vi "ADC Data capture and Process Original - Copy.vi"(0 "ADC Output Read Method":T2(ring)=enum."Read .dat file", 1 "Select the Tab to project":T1(ring)=enum."ADC Sine", 2 "ADC Input":enum16{"Sine Wave", "Ramp / Triangle"}(ring), 3 "No.of samples(SNR)":i32=4096, 4 "Resolution":i32=12, 5 "active edge":i32(ring)=10280, 6 "Inputs for Dyanmic para":T9={"Fundamental Frequency"=100000.0, "Sampling Frequncy"=3999610.0, "No of Harmonics"=9, "Window"=enum."7 Term B-Harris", "Blackman (fundamental power) bins)"=1.0}, 7 "Samples per Channel":i32=4096 caption="No.of Samples(capture)", 8 "Oversampling":bool, 9 "Oversampling ratio":i32, 10 "Drop LSB":bool, 11 "Save data":T15, 12 "Waveform":i64[](array[numeric]), 13 "Path to Read":path=path "C/Users/a0230227/Desktop/save.dat", 14 "Start & Stop Bit":cluster{"Start":i32, "Stop":i32}={"Start"=40, "Stop"=4055}, 15 "length":i32=4096, 17 "Set_Freq":dbl=100017.0, 24 "path to save":T14={"Path to Save plot"=path "D/Tenor_176P/DYN_PAR_C004/DAT/D001_TEMPP30C_VDD1.2_VDDA3.3_16B_SE_ADCA__vicA_aggX_PLT_CAP_200821_1740_33.jpg", "Path to Raw Data plot"=path "D/Tenor_176P/DYN_PAR_C004/DAT/D001_TEMPP30C_VDD1.2_VDDA3.3_16B_SE_ADCA__vicA_aggX_RAW_DAT_200821_1740_33.csv"}) -> (18 "Min Max":T4, 19 "detected Throughput":dbl, 20 "output cluster":T7, 21 "Dynamic Parameters":T8, 22 "max code":ext, 23 "min code":ext, 25 "Valid Capture":bool)   [LabVIEW 2019] (continued)
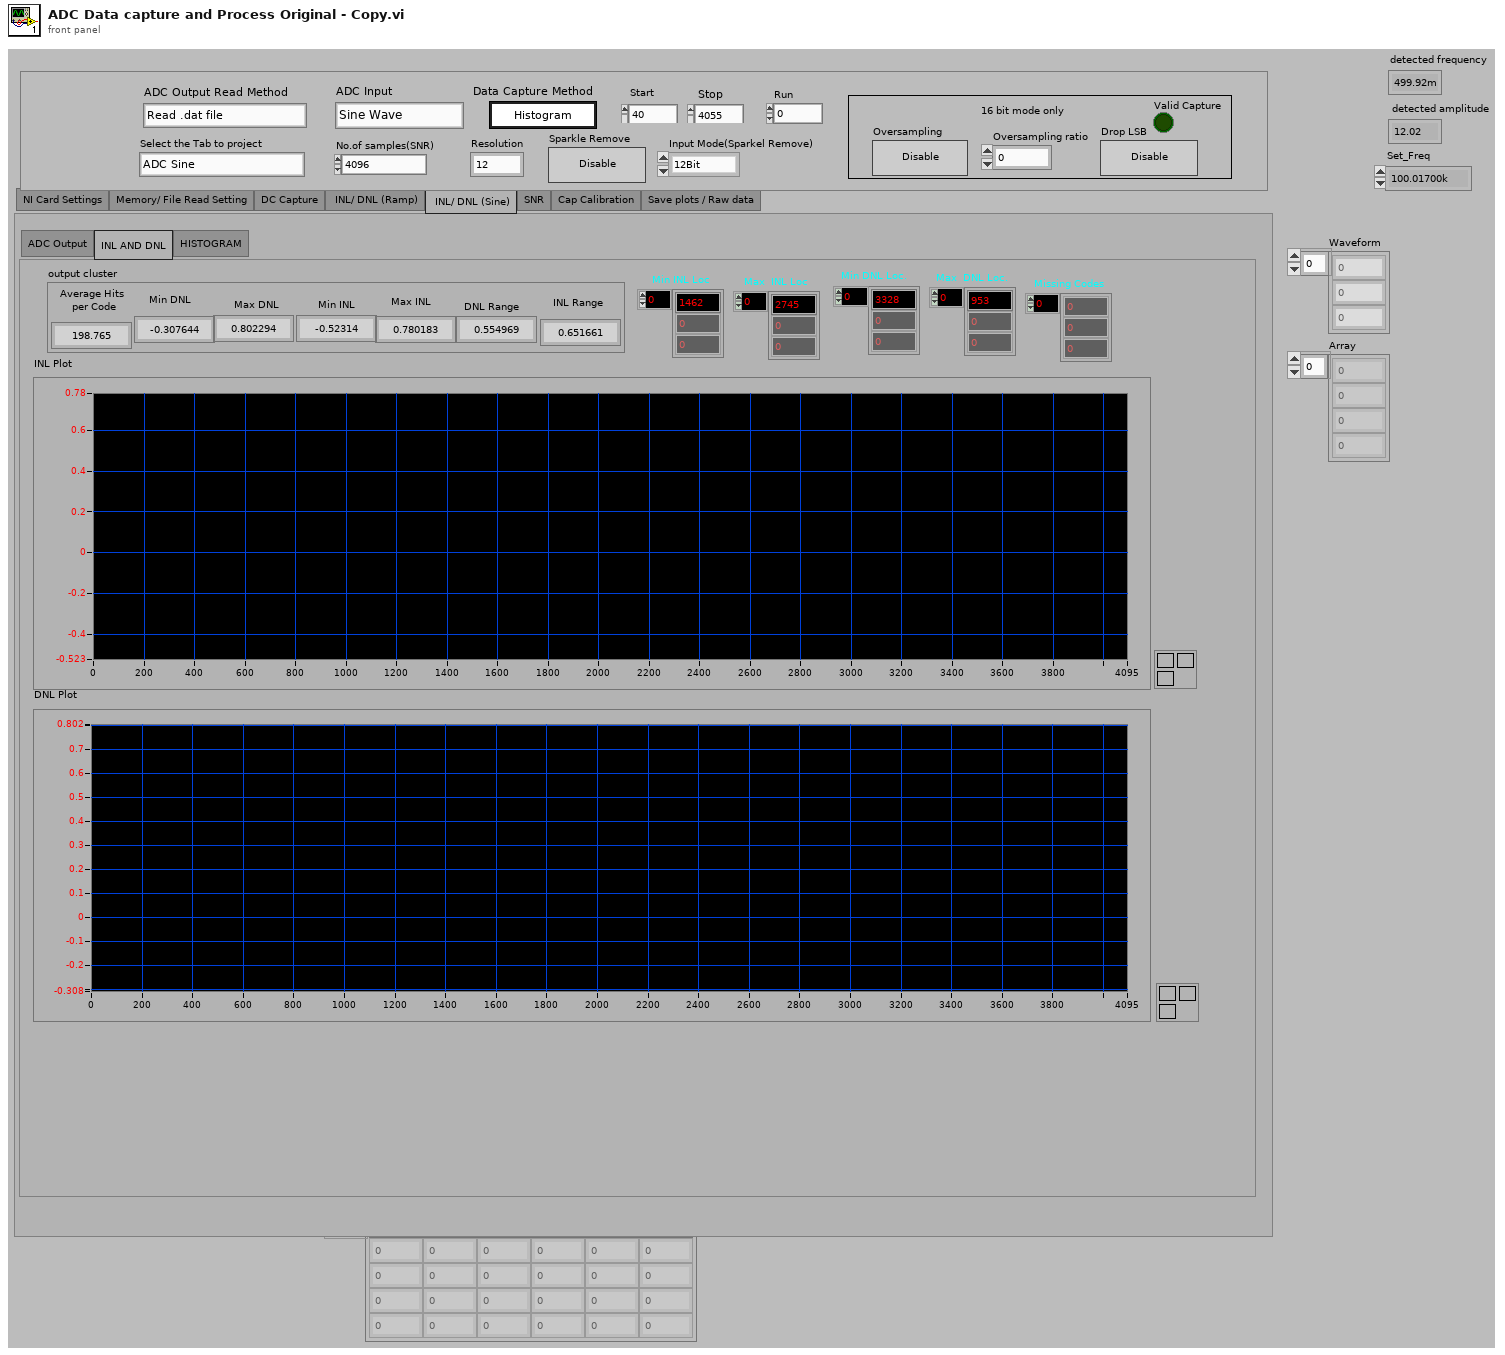
[diagram p1: front panel]
types:
  T1 = enum32{"NI Card Settings", "Memory Read Setting", "DC Capture", "ADC Ramp", "ADC Sine", "SNR", "Cap Calibration"}
  T2 = enum32{"Read from Memory", "Read .dat file", "NI Card Capture", "None"}
  T3 = enum32{"NI Card Settings", "Memory/ File Read Setting", "DC Capture", " INL/ DNL (Ramp)", " INL/ DNL (Sine)", "SNR", "Cap Calibration", "Save plots / Raw data"}
  T4 = cluster{"Min":dbl, "Max":dbl, "delta":dbl, "Average Code":dbl, "Standard Deviation":dbl}
  T5 = cluster{"Min INL":dbl, "Max INL":dbl, "Min DNL":dbl, "Max DNL":dbl, "INL Range":dbl, "DNL Range":dbl, "Avg Hits/Code":dbl}
  T6 = enum32{"ADC Output", "TRIMMED DATA", "INL AND DNL", "HISTOGRAM"}
  T7 = cluster{"Average Hits \nper Code ":dbl, "Min DNL":dbl, "Min INL":dbl, "Max INL":dbl, "Max DNL":dbl, "DNL Range":dbl, "INL Range":dbl}
  T8 = cluster{"SNR":dbl, "SNRD":dbl, "THD":dbl, "ENOB (SNRD)":dbl, "SFDR":dbl, "ENOB (SNR)":dbl, "Noise Power":dbl, "Signal power":dbl}
  T9 = cluster{"Fundamental Frequency":dbl, "Sampling Frequncy":dbl, "No of Harmonics":u8, "Window":enum16{"None ", "Hanning", "Hamming", "Blackman-Harris", "Exact Blackman", "Blackman", "Flat Top", "4 Term B-Harris ", "7 Term B-Harris"}, "Blackman (fundamental power) bins)":dbl}
  T10 = enum32{"ADC Output", "FFT Magnitude plot", " FFT plot"}
  T11 = cluster{"Ideal Power Bin":dbl, "Actual Power Bin":dbl, "Signal Strength (dB)":dbl}
  T12 = cluster{"ADC Reference(V)":dbl, "Bin Width":dbl, "PSRR/ CMRR  ":bool}
  T13 = cluster{"Fundamental Frequnecy (Calculated)":dbl, "Harmonic Frequencies":dbl[], "Harmonic Amplitudes":dbl[]}
  T14 = cluster{"Path to Save plot":path, "Path to Raw Data plot":path}
  T15 = cluster{"Save INL/DNL Plot(Ramp)":bool, "Save SNR Plot":bool, "Save INL/DNL Plot(Sine)":bool, "Save INL/DNL Raw Data(Ramp)":bool, "Save SNR Raw Data":bool, "Save INL/DNL Raw Data(Sine)":bool, "Save DC Raw data":bool, "Save  Raw Data(Sine)":bool}
  T16 = enum16{"Initialize", "Read output", "Post process", "Cap Calib", "Save data", "Exit"}
  T17 = cluster{"Average Hits \nper Code ":dbl, "Min\nDNL":dbl, dbl, dbl, "Max\nDNL":dbl, dbl, dbl}
  T18 = enum16{"None ", "Hanning", "Hamming", "Blackman-Harris", "Exact Blackman", "Blackman", "Flat Top", "4 Term B-Harris ", "7 Term B-Harris"}
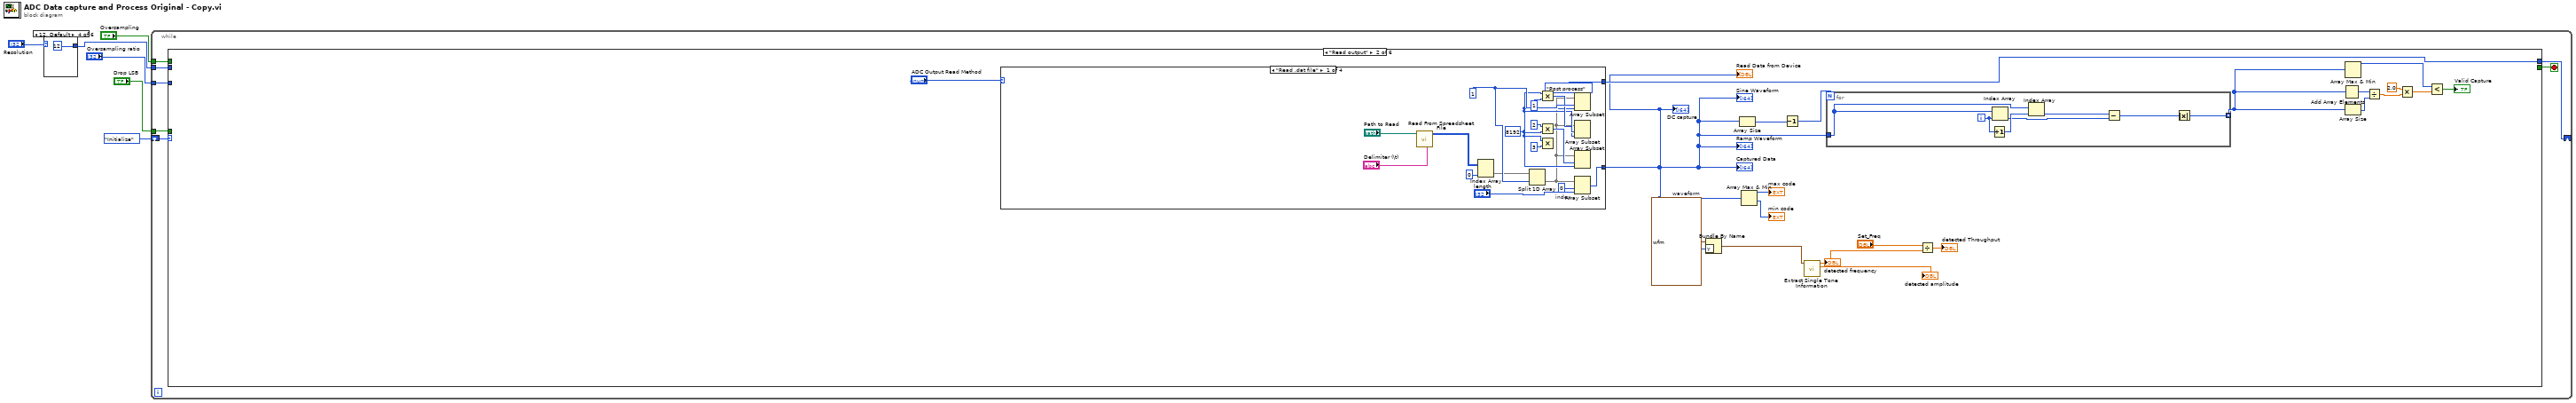
[diagram p0: block diagram]
diagram:
  n1 = case shown="12, Default" "Resolution" {
    tunnel: [18 16 14 12 10 8] -> w5
    frame 18 {
    }
    frame 16 {
    }
    frame 14 {
    }
    frame 12, Default {
    }
    frame 10 {
    }
    frame 8 {
    }
  }
  n2 = while {
    shift-right: [w18] -> _
    shift-left: T16."Initialize" -> [w19]
    tunnel: w5 -> [w16]
    tunnel: "Oversampling" -> [w15]
    tunnel: "Drop LSB" -> [w14]
    tunnel: "Oversampling ratio" -> [w13]
    stop <- w17 stop-if-true
    n3 = case shown="\"Read output\"" w19 {
      tunnel: [T16."Read output" w42 w125 T16."Save data" T16."Exit" _] -> w18
      tunnel: [_ _ _ _ _ TRUE] -> w17
      tunnel: w16 -> [_ _ w132 _ _ _]
      tunnel: w15 -> [_ _ w122 _ _ _]
      tunnel: w14 -> [_ _ w124 _ _ _]
      tunnel: w13 -> [_ _ w123 _ _ _]
      frame "Initialize", Default {
        n4 = local read "No.of samples(SNR)"() -> (w20:i32)
        n5 = local write "Samples per Channel"(w20) -> ()
      }
      frame "Read output" {
        w27 = waveform(i64) {"t0"=timestamp(0 s since 1904-01-01), "dt"=1.0, "Y"=[]}  # waveform
        n6 = case shown="\"Read .dat file\"" "ADC Output Read Method" {
          tunnel: [w52 _ w71 "Waveform"] -> w28
          tunnel: [T16."Post process" _ T16."Post process" T16."Post process"] -> w42
          frame "Read .dat file" {
            w51 = 0  # index
            w57 = 8192 ("index")
            w62 = 1 ("index")
            n7 = call-poly <vilib>:"Read From Spreadsheet File.vi"("delimiter (\\t)"="Delimiter (\\t)", "file path (dialog if empty)"="Path to Read") -> ("all rows"=w64:i64[][])  [unwired: 5 in, 4 out]
            n8 = Index Array(array=w64, index (col)=0 ("disabled index (col)")) -> (element=w55:i64[])  [unwired: 1 in]
            n9 = Split 1D Array(array=w55, index=w62) -> (second subarray=w53:i64[])  [unwired: 1 out]
            n10 = Multiply(x=w57, y=1) -> (x*y=w60:i32)
            n11 = Multiply(x=2 ("y"), y=w57) -> (x*y=w58:i32)
            n12 = Multiply(x=w57, y=3) -> ()  [unwired: 1 out]
            n13 = Array Subset(array=w53, index=w62, length=w57) -> ()  [unwired: 1 out]
            n14 = Array Subset(array=w53, index=w60, length=w57) -> ()  [unwired: 1 out]
            n15 = Array Subset(array=w53, index=w58, length=w57) -> ()  [unwired: 1 out]
            n16 = Array Subset(array=w53, index=w51, length="length") -> (w52:i64[])
          }
          frame "None" {
          }
          frame "NI Card Capture", Default {
            n17 = case shown="\"Sine Wave\", Default" "ADC Input" {
              tunnel: "Port" -> [w88 w108]
              tunnel: "Source" -> [w87 w107]
              tunnel: "Rate" -> [w86 w106]
              tunnel: "Timeout" -> [w85 w105]
              tunnel: [_ w103] -> w70
              tunnel: [w81 w104] -> w71
              tunnel: "No.of samples(SNR)" -> [w84 w102]
              tunnel: "Samples per Channel" -> [w82 w101]
              tunnel: "Sparkle Remove" -> [w80 _]
              tunnel: "active edge" -> [w79 w99]
              frame "Sine Wave", Default {
                n18 = disable-structure shown="Disabled" {
                  disable-tunnel: w88 -> [w98 _]
                  disable-tunnel: w87 -> [w97 _]
                  disable-tunnel: w86 -> [w96 _]
                  disable-tunnel: w85 -> [w95 _]
                  disable-tunnel: w84 -> [w94 _]
                  disable-tunnel: FALSE ("Histogram Capture Method SNR") -> [w93 _]
                  disable-tunnel: w82 -> [w92 _]
                  disable-tunnel: [w91 _] -> w81
                  disable-tunnel: w80 -> [w90 _]
                  disable-tunnel: w79 -> [w89 _]
                  frame Disabled {
                    n19 = call "DATA_CAPTURE_SNR.vi"("Port"=w98, "Source"=w97, "No. of samples to process"=w94, "Samples per Channel"=w92, "Rate"=w96, "active edge"=w89, "timeout"=w95, "Histogram Capture Method SNR"=w90, "NI card Cont/Single Capture"=w93) -> ("Waveform"=w91:u32[])  [unwired: 5 in, 5 out]
                  }
                  frame Enabled {
                  }
                }
              }
              frame "Ramp / Triangle" {
                n20 = disable-structure shown="Disabled" {
                  disable-tunnel: w108 -> [w119 _]
                  disable-tunnel: w107 -> [w118 _]
                  disable-tunnel: w106 -> [w117 _]
                  disable-tunnel: w105 -> [w116 _]
                  disable-tunnel: [w115 _] -> w104
                  disable-tunnel: [w114 _] -> w103
                  disable-tunnel: w102 -> [w113 _]
                  disable-tunnel: w101 -> [w111 _]
                  disable-tunnel: FALSE ("Histogram Capture Method SNR") -> [w110 _]
                  disable-tunnel: w99 -> [w109 _]
                  frame Disabled {
                    n21 = call "DATA_CAPTURE_SNR.vi"("Port"=w119, "Source"=w118, "No. of samples to process"=w113, "Samples per Channel"=w111, "Rate"=w117, "active edge"=w109, "timeout"=w116, "Histogram Capture Method SNR"=w110, "NI card Cont/Single Capture"=FALSE ("Histogram Capture Method SNR")) -> ("Waveform"=w115:u32[], "Trimmed Wave"=w114:u32[])  [unwired: 5 in, 4 out]
                  }
                  frame Enabled {
                  }
                }
              }
            }
            "Trimmed Wave" <- w70
          }
          frame "Read from Memory" {
          }
        }
        "Ramp Waveform" <- w28
        "Sine Waveform" <- w28
        "Read Data from Device" <- w28
        "Captured Data" <- w28
        "DC capture" <- w28
        n22 = Bundle By Name(cluster=w27, "Y"=w28) -> (w26:waveform(i64))
        n23 = Array Size(array=w28) -> (size(s)=w38:i32)
        n24 = Array Max & Min(array=w28) -> (max value=→"max code":i64, min value=→"min code":i64)  [unwired: 2 out]
        n25 = Decrement(x=w38) -> (x-1=w37:i32)
        n26 = call-poly <vilib>:"Extract Single Tone Information.vi"("time signal in"=w26) -> ("detected amplitude"=→"detected amplitude":dbl, "detected frequency"=w23:dbl)  [unwired: 5 in, 4 out]
        "detected frequency" <- w23
        n27 = for {
          N: w37 -> [_]
          tunnel: w28 -> [w49]
          tunnel: [w43] -> w35 mode=indexing
          i -> [w47]
          n28 = Increment(x=w47) -> (x+1=w48:i32)
          n29 = Index Array(array=w49, index=w47) -> (element=w45:i64)
          n30 = Index Array(array=w49, index=w48) -> (element=w46:i64)
          n31 = Subtract(x=w46, y=w45) -> (x-y=w44:i64)
          n32 = Absolute Value(x=w44) -> (abs(x)=w43:i64)
        }
        n33 = Divide(x="Set_Freq", y=w23) -> (x/y=→"detected Throughput":dbl)
        n34 = Add Array Elements(numeric array=w35) -> (sum=w33:i64)
        n35 = Array Max & Min(array=w35) -> (max value=w30:i64)  [unwired: 3 out]
        n36 = Array Size(array=w35) -> (size(s)=w32:i32)
        n37 = Divide(x=w33, y=w32) -> (x/y=w34:dbl)
        n38 = Multiply(x=2.0, y=w34) -> (x*y=w29:dbl)
        n39 = Less?(x=w30, y=w29) -> (x < y?=→"Valid Capture":bool)
      }
      frame "Post process" {
        n40 = local read "Select the Tab to project"() -> (w138:T1)
        n41 = local read "Read Data from Device"() -> (w129:dbl[])
        n42 = local read "No.of samples(SNR)"() -> (w131:i32)
        n43 = Equal?(x=w138, y=T1."Cap Calibration" ("Select the Tab to project")) -> (x = y?=w139:bool)
        n44 = Unbundle By Name("Start & Stop Bit") -> ("Start"=w134:i32, "Stop"=w133:i32)
        n45 = Select(t=T1."ADC Sine" ("Select the Tab to project"), s=w139, f=w138) -> (s? t:f=w137:T1)
        n46 = case shown="\"SNR\"" w137 {
          tunnel: w129 -> [w144 w260 w332 w397]
          tunnel: "Data Capture Method" -> [w141 w258 w365 _]
          tunnel: w134 -> [_ w257 w364 _]
          tunnel: w133 -> [_ w256 w363 _]
          tunnel: w132 -> [_ w259 w362 w396]
          tunnel: w131 -> [_ _ _ w398]
          tunnel: [_ w255 w350 _] -> w130
          tunnel: [T16."Save data" T16."Save data" T16."Cap Calib" T16."Save data"] -> w125
          tunnel: w122 -> [_ _ w329 w394]
          tunnel: w124 -> [_ _ w328 w393]
          tunnel: w123 -> [_ _ w330 w392]
          frame "DC Capture", Default {
            n47 = property on="Raw Data CH2" class="Arr (strict)"("Visible"="CH Swtich (To see other CH O/P)") -> ()  [unwired: 2 in, 2 out]
            n48 = property on="Standard Deviation (CH2)" class="DigNum (strict)"("Visible"="CH Swtich (To see other CH O/P)") -> ()  [unwired: 2 in, 2 out]
            n49 = property on="Raw Data CH1" class="Arr (strict)"("Visible"="CH Swtich (To see other CH O/P)") -> ()  [unwired: 2 in, 2 out]
            n50 = property on="Average Code (CH2)" class="DigNum (strict)"("Visible"="CH Swtich (To see other CH O/P)") -> ()  [unwired: 2 in, 2 out]
            n51 = case shown="False" w141 {
              tunnel: w144 -> [w147 w215]
              tunnel: "CH Swtich (To see other CH O/P)" -> [w146 _]
              tunnel: [w145 w201] -> w140
              frame False {
                n52 = case shown="True" w146 {
                  tunnel: w147 -> [w152 w189]
                  tunnel: [w148 w181] -> w145
                  frame True {
                    w158 = 10 ("index")
                    w171 = 10 ("index")
                    n53 = Decimate 1D Array(w152) -> (w168:dbl[], w159:dbl[])
                    "Raw Data CH2" <- w168
                    "Raw Data CH1" <- w159
                    n54 = Split 1D Array(array=w168, index=w171) -> (second subarray=w170:dbl[])  [unwired: 1 out]
                    n55 = Split 1D Array(array=w159, index=w158) -> (second subarray=w167:dbl[])  [unwired: 1 out]
                    n56 = Array Size(array=w170) -> (size(s)=w172:i32)
                    n57 = Array Size(array=w167) -> (size(s)=w166:i32)
                    n58 = Subtract(x=w172, y=w171) -> (x-y=w175:i32)
                    n59 = Subtract(x=w166, y=w158) -> (x-y=w156:i32)
                    n60 = Split 1D Array(array=w170, index=w175) -> (first subarray=w174:dbl[])  [unwired: 1 out]
                    n61 = Split 1D Array(array=w167, index=w156) -> (first subarray=w164:dbl[])  [unwired: 1 out]
                    n62 = Array Size(array=w174) -> (size(s)=w173:i32)
                    n63 = Array Size(array=w164) -> (size(s)=w165:i32)
                    n64 = To Double Precision Float(number=w174) -> (double precision float=w176:dbl[])
                    n65 = To Double Precision Float(number=w164) -> (double precision float=w155:dbl[])
                    n66 = Add Array Elements(numeric array=w176) -> (sum=w180:dbl)
                    n67 = Add Array Elements(numeric array=w155) -> (sum=w160:dbl)
                    n68 = Divide(x=w180, y=w173) -> (x/y=w153:dbl)
                    "Average Code (CH2)" <- w153
                    n69 = Divide(x=w160, y=w165) -> (x/y=w150:dbl)
                    n70 = Subtract(x=w176, y=w153) -> (x-y=w179:dbl[])
                    n71 = Subtract(x=w155, y=w150) -> (x-y=w161:dbl[])
                    n72 = Square(x=w179) -> (x^2=w178:dbl[])
                    n73 = Square(x=w161) -> (x^2=w162:dbl[])
                    n74 = Add Array Elements(numeric array=w178) -> (sum=w177:dbl)
                    n75 = Add Array Elements(numeric array=w162) -> (sum=w163:dbl)
                    n76 = Divide(x=w177, y=w173) -> (x/y=w169:dbl)
                    n77 = Divide(x=w163, y=w165) -> (x/y=w157:dbl)
                    n78 = Square Root(x=w169) -> (sqrt(x)=→"Standard Deviation (CH2)":dbl)
                    n79 = Square Root(x=w157) -> (sqrt(x)=w149:dbl)
                    n80 = local read "Min Max"() -> (w151:T4)
                    n81 = Bundle By Name(cluster=w151, "Average Code"=w150, "Standard Deviation"=w149) -> (w148:T4)
                  }
                  frame False {
                    w193 = 10 ("index")
                    n82 = Split 1D Array(array=w189, index=w193) -> (second subarray=w200:dbl[])  [unwired: 1 out]
                    n83 = Array Size(array=w200) -> (size(s)=w199:i32)
                    n84 = Subtract(x=w199, y=w193) -> (x-y=w191:i32)
                    n85 = Split 1D Array(array=w200, index=w191) -> (first subarray=w188:dbl[])  [unwired: 1 out]
                    n86 = Array Size(array=w188) -> (size(s)=w198:i32)
                    n87 = To Double Precision Float(number=w188) -> (double precision float=w190:dbl[])
                    n88 = Add Array Elements(numeric array=w190) -> (sum=w194:dbl)
                    n89 = Divide(x=w194, y=w198) -> (x/y=w183:dbl)
                    n90 = Subtract(x=w190, y=w183) -> (x-y=w195:dbl[])
                    n91 = Square(x=w195) -> (x^2=w196:dbl[])
                    n92 = Add Array Elements(numeric array=w196) -> (sum=w197:dbl)
                    n93 = Divide(x=w197, y=w198) -> (x/y=w192:dbl)
                    n94 = Array Max & Min(array=w188) -> (max value=w185:dbl, min value=w184:dbl)  [unwired: 2 out]
                    n95 = local read "Min Max"() -> (w187:T4)
                    n96 = Subtract(x=w185, y=w184) -> (x-y=w186:dbl)
                    n97 = Square Root(x=w192) -> (sqrt(x)=w182:dbl)
                    n98 = Bundle By Name(cluster=w187, "Standard Deviation"=w182, "Average Code"=w183, "Max"=w185, "Min"=w184, "delta"=w186) -> (w181:T4)
                  }
                }
              }
              frame True {
                n99 = for {
                  tunnel: w215 -> [w248] mode=indexing
                  shift-right: [w252] -> w224
                  shift-left: 0.0 ("x*y") -> [w253]
                  tunnel: w215 -> [w251]
                  tunnel: [w250] -> w223
                  shift-right: [w239] -> _
                  shift-left: TRUE ("x != 0?") -> [w246]
                  shift-right: [w242] -> w206
                  shift-left: i32[] [] -> [w243]
                  i -> [w245]
                  n100 = Add Array Elements(numeric array=w251) -> (sum=w250:dbl)
                  n101 = Not Equal To 0?(x=w248) -> (x != 0?=w247:bool)
                  n102 = Multiply(x=w248, y=w245) -> (x*y=w249:dbl)
                  n103 = Build Array (concatenate)(w243, w245) -> (w244:i32[])
                  n104 = And(x=w246, y=w247) -> (x .and. y?=w241:bool)
                  n105 = Add(x=w253, y=w249) -> (x+y=w252:dbl)
                  n106 = Select(t=w244, s=w241, f=w243) -> (s? t:f=w242:i32[])
                  n107 = Select(t=FALSE ("x != 0?"), s=w241, f=TRUE ("x != 0?")) -> (s? t:f=w239:bool)
                }
                n108 = Divide(x=w224, y=w223) -> (x/y=w202:dbl)
                n109 = Array Size(array=w206) -> (size(s)=w204:i32)
                n110 = Index Array(array=w206, index=0) -> (element=w207:i32)
                n111 = Split 1D Array(array=w215, index=w207) -> (second subarray=w210:dbl[])  [unwired: 1 out]
                n112 = Subtract(x=w204, y=15 ("x")) -> (x-y=w203:i32)
                n113 = Array Max & Min(array=w210) -> (max index (indices)=w218:i32)  [unwired: 3 out]
                n114 = Greater?(x=w218, y=w203) -> (0:w219:bool)
                n115 = case shown="True" w219 {
                  tunnel: w218 -> [w227 w234]
                  tunnel: [w226 w234] -> w214
                  tunnel: 10 ("y") -> [w231 w233]
                  tunnel: w210 -> [w230 w237]
                  tunnel: [w227 w236] -> w213
                  tunnel: [_ w232] -> w208
                  frame True {
                    n116 = Subtract(x=w227, y=w231) -> (x-y=w228:i32)
                    n117 = Split 1D Array(array=w230, index=w228) -> (first subarray=w229:dbl[])  [unwired: 1 out]
                    n118 = Array Max & Min(array=w229) -> (max index (indices)=w226:i32)  [unwired: 3 out]
                  }
                  frame False {
                    n119 = Add(x=w234, y=w233) -> (x+y=w232:i32)
                    n120 = Split 1D Array(array=w237, index=w232) -> (second subarray=w235:dbl[])  [unwired: 1 out]
                    n121 = Array Max & Min(array=w235) -> (max index (indices)=w236:i32)  [unwired: 3 out]
                  }
                }
                n122 = Add(x=w207, y=w214) -> (x+y=w211:i32)
                n123 = Compound Arithmetic op=ADD(w207, w213, w208) -> (w212:i32)
                n124 = Subtract(x=w212, y=w211) -> (x-y=w217:i32)
                n125 = local read "Min Max"() -> (w222:T4)
                n126 = Bundle By Name(cluster=w222, "Average Code"=w202, "Min"=w211, "Max"=w212, "delta"=w217) -> (w201:T4)
              }
            }
            "Min Max" <- w140
          }
          frame "ADC Ramp" {
            n127 = stacked-sequence {
              seq-local: [w262 _ _] -> [_ w286 _]
              seq-local: [_ w282 _] -> [_ _ w312]
              seq-local: [_ w281 _] -> [_ _ w311]
              seq-local: [_ w280 _] -> [_ _ w300]
              seq-local: [w263 _ _] -> [_ w279 _]
              tunnel: w260 -> [w265 _ _]
              tunnel: w259 -> [w267 _ _]
              tunnel: w258 -> [w266 _ _]
              tunnel: w257 -> [_ w285 _]
              tunnel: w256 -> [_ w284 _]
              tunnel: [w262 _ _] -> w255
              frame #0 {
                n128 = local read "Trimmed Wave"() -> (w261:u32[])
                n129 = Scale By Power Of 2(n=w267, x=ext 1.0) -> (x*2^n=w263:ext)
                n130 = Initialize Array(0 ("element"), w263) -> (w271:i32[])
                n131 = for {
                  shift-right: [w274] -> w264
                  shift-left: w271 -> [w275]
                  tunnel: 0.0 -> [w273]
                  tunnel: w261 -> [w272] mode=indexing
                  n132 = Subtract(x=w272, y=w273) -> (x-y=w276:dbl)
                  n133 = in-place {
                    n134 = in-place-array #1(w275, w276) -> (w278:i32)
                    n135 = Increment(x=w278) -> (x+1=w277:i32)
                    n136 = in-place-array #1(w277) -> (w274:i32[])  [unwired: 1 out]
                  }
                }
                n137 = Select(t=w265, s=w266, f=w264) -> (s? t:f=w262:dbl[])
                "Histogram waveform" <- w262
              }
              frame #1 {
                n138 = Subtract(x=w284, y=w285) -> (x-y=w287:i32)
                n139 = Split 1D Array(array=w286, index=w285) -> (second subarray=w294:dbl[])  [unwired: 1 out]
                n140 = Split 1D Array(array=w294, index=w287) -> (first subarray=w288:dbl[])  [unwired: 1 out]
                n141 = Add Array Elements(numeric array=w288) -> (sum=w291:dbl)
                n142 = Array Size(array=w288) -> (size(s)=w290:i32)
                n143 = Divide(x=w291, y=w290) -> (x/y=w280:dbl)
                n144 = Initialize Array(w280, w279) -> (w289:dbl[])
                n145 = Replace Array Subset(array=w289, new element=w288, index=w285) -> (w293:dbl[])
                n146 = Divide(x=w293, y=w280) -> (x/y=w292:dbl[])
                n147 = Decrement(x=w292) -> (x-1=w282:dbl[])
                "DNL_Ramp" <- w282
                n148 = for {
                  shift-right: [w296] -> _
                  shift-left: 0.0 ("x") -> [w297]
                  tunnel: [w296] -> w281 mode=indexing
                  tunnel: w282 -> [w295] mode=indexing
                  n149 = Add(x=w297, y=w295) -> (x+y=w296:dbl)
                }
                "INL_Ramp" <- w281
              }
              frame #2 {
                n150 = Array Max & Min(array=w312) -> (max value=w303:dbl, min value=w304:dbl)  [unwired: 2 out]
                n151 = Array Max & Min(array=w311) -> (max value=w305:dbl, min value=w306:dbl)  [unwired: 2 out]
                n152 = Subtract(x=w303, y=w304) -> (x-y=w308:dbl)
                n153 = Subtract(x=w305, y=w306) -> (x-y=w309:dbl)
                n154 = local read "Static Parameters (Ramp)"() -> (w299:T5)
                n155 = Divide(x=w308, y=2.0) -> (x/y=w301:dbl)
                n156 = Divide(x=w309, y=2.0) -> (x/y=w302:dbl)
                n157 = disable-structure shown="Enabled" {
                  disable-tunnel: w306 -> [w327 _]
                  disable-tunnel: w305 -> [w326 _]
                  disable-tunnel: w304 -> [w325 _]
                  disable-tunnel: w303 -> [w324 _]
                  disable-tunnel: w302 -> [w315 _]
                  disable-tunnel: w301 -> [w314 _]
                  disable-tunnel: w300 -> [w313 _]
                  frame Disabled {
                    n158 = Increment(x="Run") -> (x+1=w316:dbl)
                    n159 = local write "Run"(w316) -> ()
                    n160 = Build Array(w316, w327, w326, w325, w324, w315, w314, w313) -> (w323:dbl[])
                    n161 = call-poly <vilib>:"Write To Spreadsheet File.vi"("delimiter (\\t)"="," ("delimiter (\\t)"), "transpose? (no:F)"=FALSE, "format (%.3f)"="%.4f", "append to file? (new file:F)"=TRUE, "1D data"=w323, "file path (dialog if empty)"=path "D:/FALCON/ADC/Raw_Data/runtorun.csv") -> ()  [unwired: 2 in, 1 out]
                  }
                  frame Enabled {
                  }
                }
                n162 = Bundle By Name(cluster=w299, "Max INL"=w305, "Min INL"=w306, "Max DNL"=w303, "Min DNL"=w304, "INL Range"=w302, "DNL Range"=w301, "Avg Hits/Code"=w300) -> (→"Static Parameters (Ramp)":T5)
              }
            }
          }
          frame "ADC Sine" {
            n163 = case shown="True" w329 {
              tunnel: w332 -> [w367 w375]
              tunnel: [w368 w373] -> w331
              tunnel: w330 -> [_ w374]
              tunnel: w328 -> [w366 _]
              frame False {
                n164 = case shown="True" w366 {
                  tunnel: w367 -> [w369 w371]
                  tunnel: [w369 w370] -> w368
                  frame False {
                  }
                  frame True {
                    n165 = Divide(x=w371, y=2.0) -> (x/y=w370:dbl[])
                  }
                }
              }
              frame True {
                n166 = Array Size(array=w375) -> (size(s)=w377:i32)
                n167 = Divide(x=w377, y=w374) -> (x/y=w376:dbl)
                n168 = for {
                  N: w376 -> [_]
                  tunnel: w375 -> [w384]
                  tunnel: w374 -> [w379]
                  tunnel: [w378] -> w373 mode=indexing
                  i -> [w383]
                  n169 = Multiply(x=w379, y=w383) -> (x*y=w382:i32)
                  n170 = Array Subset(array=w384, index=w382, length=w379) -> (w381:dbl[])
                  n171 = Add Array Elements(numeric array=w381) -> (sum=w380:dbl)
                  n172 = Divide(x=w380, y=w379) -> (x/y=w378:dbl)
                }
              }
            }
            n173 = call "Sinewave_Linearity_trial_F027.vi"("Array"=w331, "Histogram Capture Method"=w365, "L code"=w364, "UCode"=w363, "Resolution"=w362, "Histogram: h(x)"=w331) -> ("Average Hits \nper Code"=w340:dbl, "Max\nDNL"=w336:dbl, "Min\nDNL"=w339:dbl, "Missing Codes"=→"Missing Codes":i32[], "Max  DNL Loc."=→"Max  DNL Loc.":i32[], "Min DNL Loc."=→"Min DNL Loc.":i32[], "Max  INL Loc"=→"Max  INL Loc":i32[], "Min INL Loc"=→"Min INL Loc":i32[], "Histogram Plot"=w352:dbl[][], "DNL Plot"=w348:dbl[], "INL Plot"=w341:dbl[])  [unwired: 1 in, 2 out]
            "Histogram Plot" <- w352
            "DNL Plot" <- w348
            "INL Plot" <- w341
            n174 = for {
              tunnel: w348 -> [w391] mode=indexing
              tunnel: [w387] -> w347 mode=indexing
              shift-right: [w386] -> _
              shift-left: 16384 ("f") -> [w385]
              i -> [w388]
              n175 = Increment(x=w385) -> (x+1=w386:i32)
              n176 = Greater?(x=w391, y=0.9) -> (0:w389:bool)
              n177 = Select(t=w388, s=w389, f=w385) -> (s? t:f=w387:i32)
            }
            n178 = Subtract(x=w336, y=w339) -> (x-y=w359:dbl)
            n179 = Array Max & Min(array=w341) -> (max value=w337:dbl, min value=w338:dbl)  [unwired: 2 out]
            n180 = Index Array(array=w352, index (col)=1 ("disabled index (col)")) -> (element=w350:dbl[])  [unwired: 1 in]
            n181 = Subtract(x=w337, y=w338) -> (x-y=w361:dbl)
            n182 = Divide(x=w359, y=2.0) -> (x/y=w335:dbl)
            n183 = Divide(x=w361, y=2.0) -> (x/y=w334:dbl)
            n184 = Bundle("Average Hits \nper Code"=w340, "Min\nDNL"=w339, w338, w337, "Max\nDNL"=w336, w335, w334) -> (→"output cluster":T17)  [unwired: 1 in]
            n185 = Sort 1D Array(array=w347) -> (sorted array=w343:i32[])
            n186 = Search 1D Array(1D array=w343, element=16384) -> (index of element=w344:i32)  [unwired: 1 in]
            n187 = Array Subset(array=w343, length=w344) -> (→"Array":i32[])  [unwired: 1 in]
          }
          frame "SNR" {
            n188 = stacked-sequence {
              seq-local: [w419 _ _] -> [_ w480 _]
              seq-local: [w418 _ _] -> [_ _ w505]
              seq-local: [w412 _ _] -> [_ _ w508]
              seq-local: [w411 _ _] -> [_ _ w504]
              seq-local: [w410 _ _] -> [_ _ w503]
              tunnel: w398 -> [w431 _ w506]
              tunnel: w397 -> [w413 _ _]
              tunnel: w396 -> [w415 _ _]
              tunnel: w394 -> [w402 _ _]
              tunnel: w393 -> [w401 _ _]
              tunnel: w392 -> [w400 _ _]
              frame #0 {
                n189 = Unbundle By Name("PSRR/CMRR Input") -> ("ADC Reference(V)"=w414:dbl, "PSRR/ CMRR"=w410:bool)
                n190 = case shown="True" w410 {
                  tunnel: 1.0 ("x") -> [_ w466]
                  tunnel: w415 -> [_ w465]
                  tunnel: w414 -> [_ w463]
                  tunnel: w413 -> [w459 w461]
                  tunnel: [w459 w460] -> w404
                  frame False {
                  }
                  frame True {
                    n191 = Scale By Power Of 2(n=w465, x=w466) -> (x*2^n=w464:dbl)
                    n192 = Divide(x=w463, y=w464) -> (x/y=w462:dbl)
                    n193 = Multiply(x=w461, y=w462) -> (x*y=w460:dbl[])
                  }
                }
                n194 = case shown="True" w402 {
                  tunnel: w404 -> [w441 w449]
                  tunnel: [w442 w447] -> w403
                  tunnel: w400 -> [_ w448]
                  tunnel: w401 -> [w440 _]
                  frame False {
                    n195 = case shown="True" w440 {
                      tunnel: w441 -> [w443 w445]
                      tunnel: [w443 w444] -> w442
                      frame False {
                      }
                      frame True {
                        n196 = Divide(x=w445, y=2.0) -> (x/y=w444:dbl[])
                      }
                    }
                  }
                  frame True {
                    n197 = Array Size(array=w449) -> (size(s)=w451:i32)
                    n198 = Divide(x=w451, y=w448) -> (x/y=w450:dbl)
                    n199 = for {
                      N: w450 -> [_]
                      tunnel: w449 -> [w458]
                      tunnel: w448 -> [w453]
                      tunnel: [w452] -> w447 mode=indexing
                      i -> [w457]
                      n200 = Multiply(x=w453, y=w457) -> (x*y=w456:i32)
                      n201 = Array Subset(array=w458, index=w456, length=w453) -> (w455:dbl[])
                      n202 = Add Array Elements(numeric array=w455) -> (sum=w454:dbl)
                      n203 = Divide(x=w454, y=w453) -> (x/y=w452:dbl)
                    }
                  }
                }
                n204 = Unbundle By Name("Inputs for Dyanmic para") -> ("Window"=w429:T18, "Sampling Frequncy"=w418:dbl, "Fundamental Frequency"=w412:dbl, "No of Harmonics"=w419:u8, "Blackman (fundamental power) bins)"=w428:dbl)
                n205 = Reciprocal(x=w418) -> (1/x=w433:dbl)
                n206 = call-poly <vilib>:"Scaled Time Domain Window.vi"("window"=w429, "X"=w403) -> ("Windowed X"=w437:dbl[])  [unwired: 7 in, 2 out]
                n207 = local read "Dynamic Parameters"() -> (w427:T8)
                n208 = call <vilib>:"Auto Power Spectrum.vi"("dt"=w433, "Signal (V)"=w437) -> ("Power Spectrum (V^2 rms)"=w432:dbl[])  [unwired: 1 out]
                n209 = Logarithm Base 10(1:w432) -> (0:w439:dbl[])
                n210 = call "Calculate_SNR_THD.vi"("Auto Power Spectrum"=w432, "frame size"=w431, "# harmonics"=w419, "window"=w429, "sampling rate"=w418, "fundamental frequency"=w412, "Blackman\n (fundamental power bins)"=w428) -> ("% THD"=w426:dbl, "ENOB(SNRD)"=w421:dbl, "% THD + Noise"=w399:dbl, "ENOB(SNR)"=w422:dbl, "Noise Power"=w425:dbl, "Fundamental frequency Calculated"=w407:dbl, "SNR"=w424:dbl, "Signal power"=w423:dbl, "Harmonic Amplitudes"=w434:dbl[], "Harmonic Frequencies"=w409:dbl[])  [unwired: 3 in]
                n211 = Bundle By Name(cluster=w427, "THD"=w426, "SNRD"=w399, "Noise Power"=w425, "SNR"=w424, "Signal power"=w423, "ENOB (SNR)"=w422, "ENOB (SNRD)"=w421) -> (→"Dynamic Parameters":T8)
                n212 = Logarithm Base 10(1:w434) -> (0:w436:dbl[])
                n213 = Multiply(x=10.0, y=w439) -> (x*y=w411:dbl[])
                "FFT Magnitude Plot (dB)" <- w411
                n214 = local read "Harmonic Details"() -> (w405:T13)
                n215 = Multiply(x=20, y=w436) -> (x*y=w408:dbl[])
                n216 = Bundle By Name(cluster=w405, "Fundamental Frequnecy (Calculated)"=w407, "Harmonic Frequencies"=w409, "Harmonic Amplitudes"=w408) -> (→"Harmonic Details":T13)
              }
              frame #1 {
                n217 = local read "Harmonic Details"() -> (w468:T13)
                n218 = Unbundle By Name(w468) -> ("Harmonic Amplitudes"=w467:dbl[])
                n219 = Decrement(x=w480) -> (x-1=w486:u8)
                n220 = Index Array(array=w467, index=0) -> (element=w482:dbl)
                n221 = Array Subset(array=w467, index=1, length=w486) -> (w484:dbl[])
                n222 = Array Max & Min(array=w484) -> (max value=w481:dbl)  [unwired: 3 out]
                n223 = local read "Dynamic Parameters"() -> (w479:T8)
                n224 = Subtract(x=w482, y=w481) -> (x-y=w478:dbl)
                n225 = Bundle By Name(cluster=w479, "SFDR"=w478) -> (w477:T8)
                n226 = local write "Dynamic Parameters"(w477) -> ()
                n227 = Unbundle By Name(w477) -> ("SNR"=w476:dbl, "SNRD"=w475:dbl, "THD"=w474:dbl, "SFDR"=w473:dbl, "ENOB (SNR)"=w472:dbl, "ENOB (SNRD)"=w471:dbl, "Noise Power"=w470:dbl, "Signal power"=w469:dbl)
                n228 = disable-structure shown="Enabled" {
                  disable-tunnel: w476 -> [w502 _]
                  disable-tunnel: w475 -> [w501 _]
                  disable-tunnel: w471 -> [w489 _]
                  disable-tunnel: w474 -> [w492 _]
                  disable-tunnel: w473 -> [w491 _]
                  disable-tunnel: w472 -> [w490 _]
                  disable-tunnel: w470 -> [w488 _]
                  disable-tunnel: w469 -> [w487 _]
                  frame Disabled {
                    n229 = local read "Run"() -> (w493:dbl)
                    n230 = Increment(x=w493) -> (x+1=w494:dbl)
                    n231 = local write "Run"(w494) -> ()
                    n232 = Build Array(w494, w502, w501, w492, w491, w490, w489, w488, w487) -> (w500:dbl[])
                    n233 = call-poly <vilib>:"Write To Spreadsheet File.vi"("delimiter (\\t)"="," ("delimiter (\\t)"), "transpose? (no:F)"=FALSE, "format (%.3f)"="%.4f", "append to file? (new file:F)"=TRUE, "1D data"=w500, "file path (dialog if empty)"=path "D:/FALCON/ADC/Raw_Data/runtorun.csv") -> ()  [unwired: 2 in, 1 out]
                  }
                  frame Enabled {
                  }
                }
              }
              frame #2 {
                n234 = local read "FFT Magnitude Plot (dB)"() -> (w515:dbl[])
                n235 = Array Size(array=w515) -> (size(s)=w514:i32)
                n236 = Divide(x=w505, y=2.0) -> (x/y=w512:dbl)
                n237 = for {
                  N: w514 -> [_]
                  tunnel: w515 -> [w558]
                  tunnel: [w553] -> w510 mode=indexing
                  tunnel: w514 -> [w556]
                  tunnel: w512 -> [w554]
                  tunnel: [w552] -> w511 mode=indexing
                  tunnel: [w552] -> w507
                  i -> [w557]
                  n238 = Divide(x=w557, y=w556) -> (x/y=w555:dbl)
                  n239 = Index Array(array=w558, index=w557) -> (element=w553:dbl)
                  n240 = Multiply(x=w555, y=w554) -> (x*y=w552:dbl)
                }
                n241 = case shown="True" w503 {
                  tunnel: w508 -> [_ w519]
                  tunnel: w507 -> [_ w520]
                  tunnel: w506 -> [_ w534]
                  tunnel: w505 -> [_ w522]
                  tunnel: w504 -> [_ w526]
                  frame False {
                  }
                  frame True {
                    n242 = Greater?(x=w519, y=w520) -> (0:w521:bool)
                    n243 = case shown="True" w521 {
                      tunnel: [w537 w538] -> w518
                      tunnel: w519 -> [w537 w544]
                      tunnel: w522 -> [_ w543]
                      tunnel: w520 -> [_ _]
                      tunnel: w519 -> [_ w542]
                      frame False {
                      }
                      frame True {
                        n244 = while {
                          tunnel: w543 -> [w551]
                          tunnel: w544 -> [w548]
                          shift-right: [w546] -> _
                          shift-left: w543 -> [w545]
                          shift-left: w543 -> [_]
                          tunnel: [w545] -> w541
                          i -> [w549]
                          stop <- w547 continue-if-true
                          n245 = Increment(x=w549) -> (x+1=w550:i32)
                          n246 = Multiply(x=w551, y=w550) -> (x*y=w546:dbl)
                          n247 = Greater?(x=w548, y=w546) -> (0:w547:bool)
                        }
                        n248 = Subtract(x=w541, y=w542) -> (x-y=w539:dbl)
                        n249 = Sign(1:w539) -> (0:w540:dbl)
                        n250 = Multiply(x=w539, y=w540) -> (x*y=w538:dbl)
                      }
                    }
                    n251 = Multiply(x=w534, y=w518) -> (x*y=w536:dbl)
                    n252 = local read "PSRR/CMRR Input"() -> (w532:T12)
                    n253 = Divide(x=w536, y=w522) -> (x/y=w535:dbl)
                    n254 = Unbundle By Name(w532) -> ("Bin Width"=w517:dbl)
                    n255 = To Long Integer(number=w535) -> (32bit integer=w531:i32)
                    n256 = Subtract(x=w531, y=w517) -> (x-y=w527:dbl)
                    n257 = Add(x=w531, y=w517) -> (x+y=w516:dbl)
                    n258 = Split 1D Array(array=w526, index=w516) -> (first subarray=w530:dbl[])  [unwired: 1 out]
                    n259 = Split 1D Array(array=w530, index=w527) -> (second subarray=w529:dbl[])  [unwired: 1 out]
                    n260 = Array Max & Min(array=w529) -> (max value=w525:dbl, max index (indices)=w528:i32)  [unwired: 2 out]
                    n261 = local read "PSRR/CMRR Output"() -> (w533:T11)
                    n262 = Add(x=w528, y=w527) -> (x+y=w524:dbl)
                    n263 = Bundle By Name(cluster=w533, "Ideal Power Bin"=w531, "Actual Power Bin"=w524, "Signal Strength (dB)"=w525) -> (→"PSRR/CMRR Output":T11)
                  }
                }
                n264 = Bundle(w511, w510) -> (→"FFT Plot":cluster{dbl[], dbl[]})  [unwired: 1 in]
              }
            }
          }
        }
        n265 = Build Array(w129, w130) -> (→"Raw_Histo":dbl[][])
      }
      frame "Cap Calib" {
        n266 = case shown="\"64\"" "Average Window" {
          tunnel: [8 16 32 64] -> w559
          frame "8", Default {
          }
          frame "16" {
          }
          frame "32" {
          }
          frame "64" {
          }
        }
        n267 = case shown="True" "Cap Calibration" {
          tunnel: w559 -> [_ w567]
          frame False {
          }
          frame True {
            n268 = local read "DNL Plot"() -> (w568:dbl[])
            n269 = local read "INL Plot"() -> (w569:dbl[])
            n270 = disable-structure shown="Disabled" {
              disable-tunnel: "INL/DNL Values" -> [w588 _]
              disable-tunnel: "File path (DNL & INL)" -> [w587 _]
              disable-tunnel: "Select Channel" -> [w586 _]
              disable-tunnel: [w585 _] -> w574
              disable-tunnel: [w584 _] -> w573
              disable-tunnel: [w583 _] -> w572
              disable-tunnel: [w582 _] -> w571
              disable-tunnel: [w581 _] -> w570
              disable-tunnel: w569 -> [w580 _]
              disable-tunnel: w568 -> [w579 _]
              disable-tunnel: w567 -> [w578 _]
              frame Disabled {
                n271 = call "Cap_Calibration.vi"("INL"=w580, "DNL"=w579, "From File/ Waveform"=w588, "Select Channel"=w586, "Average Window"=w578, "File path (DNL & INL)"=w587) -> ("ADC TEST 7"=w581:string, "ADC TEST 6"=w582:string, "ADC TEST 5"=w583:string, "Trim Coeff (Binary)"=w585:string[], "Trim Coeff (Integer)"=w584:dbl[])  [unwired: 1 in]
              }
              frame Enabled {
              }
            }
            "Trim Coeff (Binary)" <- w574
            "Trim Coeff (Integer)" <- w573
            "ADC TEST 5" <- w572
            "ADC TEST 6" <- w571
            "ADC TEST 7" <- w570
          }
        }
      }
      frame "Save data" {
        n272 = Unbundle By Name("path to save") -> ("Path to Save plot"=w589:path, "Path to Raw Data plot"=w592:path)
        n273 = disable-structure shown="Enabled" {
          disable-tunnel: w592 -> [w613 w725]
          disable-tunnel: [w605 w725] -> w590
          frame Disabled {
            w603 = "16Hits_Run" ("regular expression")
            n274 = local read "Run"() -> (w604:dbl)
            n275 = Increment(x=w604) -> (x+1=w608:dbl)
            n276 = local write "Run"(w608) -> ()
            n277 = Path To String(path=w613) -> (string=w612:string)
            n278 = Number To Decimal String(number=w608) -> (decimal integer string=w609:string)  [unwired: 1 in]
            n279 = xnode "Match Regular Expression"("input string"=w612, "regular expression"=w603) -> ("before match"=w611:string, "after match"=w610:string)  [unwired: 4 in, 3 out]
            n280 = Concatenate Strings(w603, w609) -> (w607:string)
            n281 = Concatenate Strings(w611, w607, w610) -> (w606:string)
            n282 = String To Path(string=w606) -> (path=w605:path)
          }
          frame Enabled {
          }
        }
        n283 = Unbundle By Name("Save data") -> ("Save INL/DNL Plot(Ramp)"=w599:bool, "Save INL/DNL Raw Data(Ramp)"=w598:bool, "Save INL/DNL Plot(Sine)"=w597:bool, "Save INL/DNL Raw Data(Sine)"=w596:bool, "Save SNR Plot"=w595:bool, "Save SNR Raw Data"=w594:bool, "Save DC Raw data"=w591:bool)  [unwired: 1 out]
        n284 = case shown="\"ADC Ramp\"" "Select the Tab to project" {
          tunnel: w589 -> [w729 w749 w773 _ _]
          tunnel: w590 -> [w730 w750 w772 _ w789]
          tunnel: w599 -> [w727 _ _ _ _]
          tunnel: w598 -> [w726 _ _ _ _]
          tunnel: w597 -> [_ w747 _ _ _]
          tunnel: w596 -> [_ w746 _ _ _]
          tunnel: w595 -> [_ _ w770 _ _]
          tunnel: w594 -> [_ _ w769 _ _]
          tunnel: w591 -> [_ _ _ _ w788]
          frame "ADC Ramp" {
            n285 = case shown="True" w727 {
              tunnel: w729 -> [_ w732]
              frame False {
              }
              frame True {
                n286 = Current VI's Path() -> (path=w733:path)
                n287 = call "Take fron panel screenshot.vi"("VI path"=w733, "Image path"=w732, "Visible area only? (f)"=FALSE, "File type (.jpg)"=enum16{".bmp", ".png", ".jpg"}.".png") -> ()  [unwired: 4 in, 1 out]
              }
            }
            n288 = case shown="True" w726 {
              tunnel: w730 -> [_ w739]
              frame False {
              }
              frame True {
                w738 = "" ("delimiter (\\t)")
